vi "StartCaller.vi"   [LabVIEW 2013]
uses:
  Counter.lvclass/Counter.lvclass
  <vilib>/ActorFramework/Message Queue/Message Queue.lvclass/Message Queue.ctl
  <vilib>/ActorFramework/Message Queue/Message Queue.lvclass
  <vilib>/ActorFramework/Actor/Actor.lvclass
panel:
  # "Start To Run"
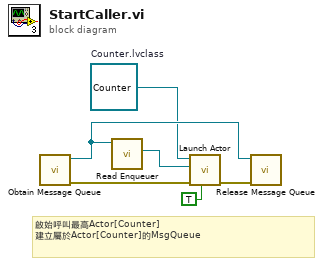
[diagram p0: block diagram]
diagram:
  w2 = refnum<class "Counter.lvclass"> refnum  # Counter.lvclass
  # "啟始呼叫最高Actor[Counter]\n建立屬於Actor[Counter]的MsgQueue"
  n1 = call <vilib>:"Obtain Message Queue.vi"() -> ("error out"=w5:errorcluster, "Message Queue"=w3:refnum<class "Message Queue.lvclass">)  [unwired: 10 in]
  n2 = call <vilib>:"Read Enqueuer.vi"("Message Queue"=w3) -> ("Message Enqueuer"=w6:refnum<class "Message Enqueuer.lvclass">)  [unwired: 10 in]
  n3 = call <vilib>:"Launch Actor.vi"("Open Actor Core front panel? (F)"=TRUE, "error in (no error)"=w5, "Actor-to-Caller Enqueuer"=w6, "Actor"=w2) -> ("error out"=w1:errorcluster)  [unwired: 6 in, 1 out]
  n4 = call <vilib>:"Release Message Queue.vi"("error in (no error)"=w1, "Message Queue"=w3) -> ()  [unwired: 8 in, 2 out]
